vi "SimulationEngine-Media.vi"(0 "Use Slab Geometry (F: Sphere)":bool, 1 "File Prefix":string, 4 "Simulation Grain (mm)":dbl=0.0001, 5 "Radius (mm)":dbl=5.0, 6 "N Photons":i32=1, 7 "Starting Depth (mm)":dbl=2.0, 8 "G":dbl=nan, 9 "Absorption Coefficient":dbl=0.00645, 10 "Scattering Coefficient":dbl=1.688, 11 "folder path":path) -> (2 "Diagram":cluster{dbl[], dbl[]}[](graph), 3 "new file path (Not A Path if cancelled)":path)   [LabVIEW 2019]
uses:
  <vilib>/Utility/file.llb/Write Delimited Spreadsheet (string).vi
panel:
  out "Numeric":i32
  out "dT":dbl
  out "Current Index":i32
  # "18.638"
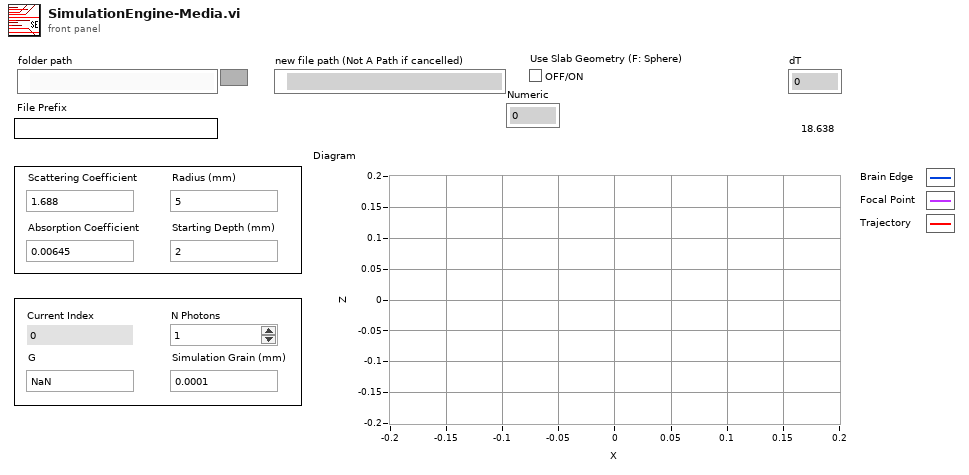
[diagram p1: front panel]
types:
  T1 = cluster{"Starting Depth":dbl, "Starting Depth":dbl, dbl}
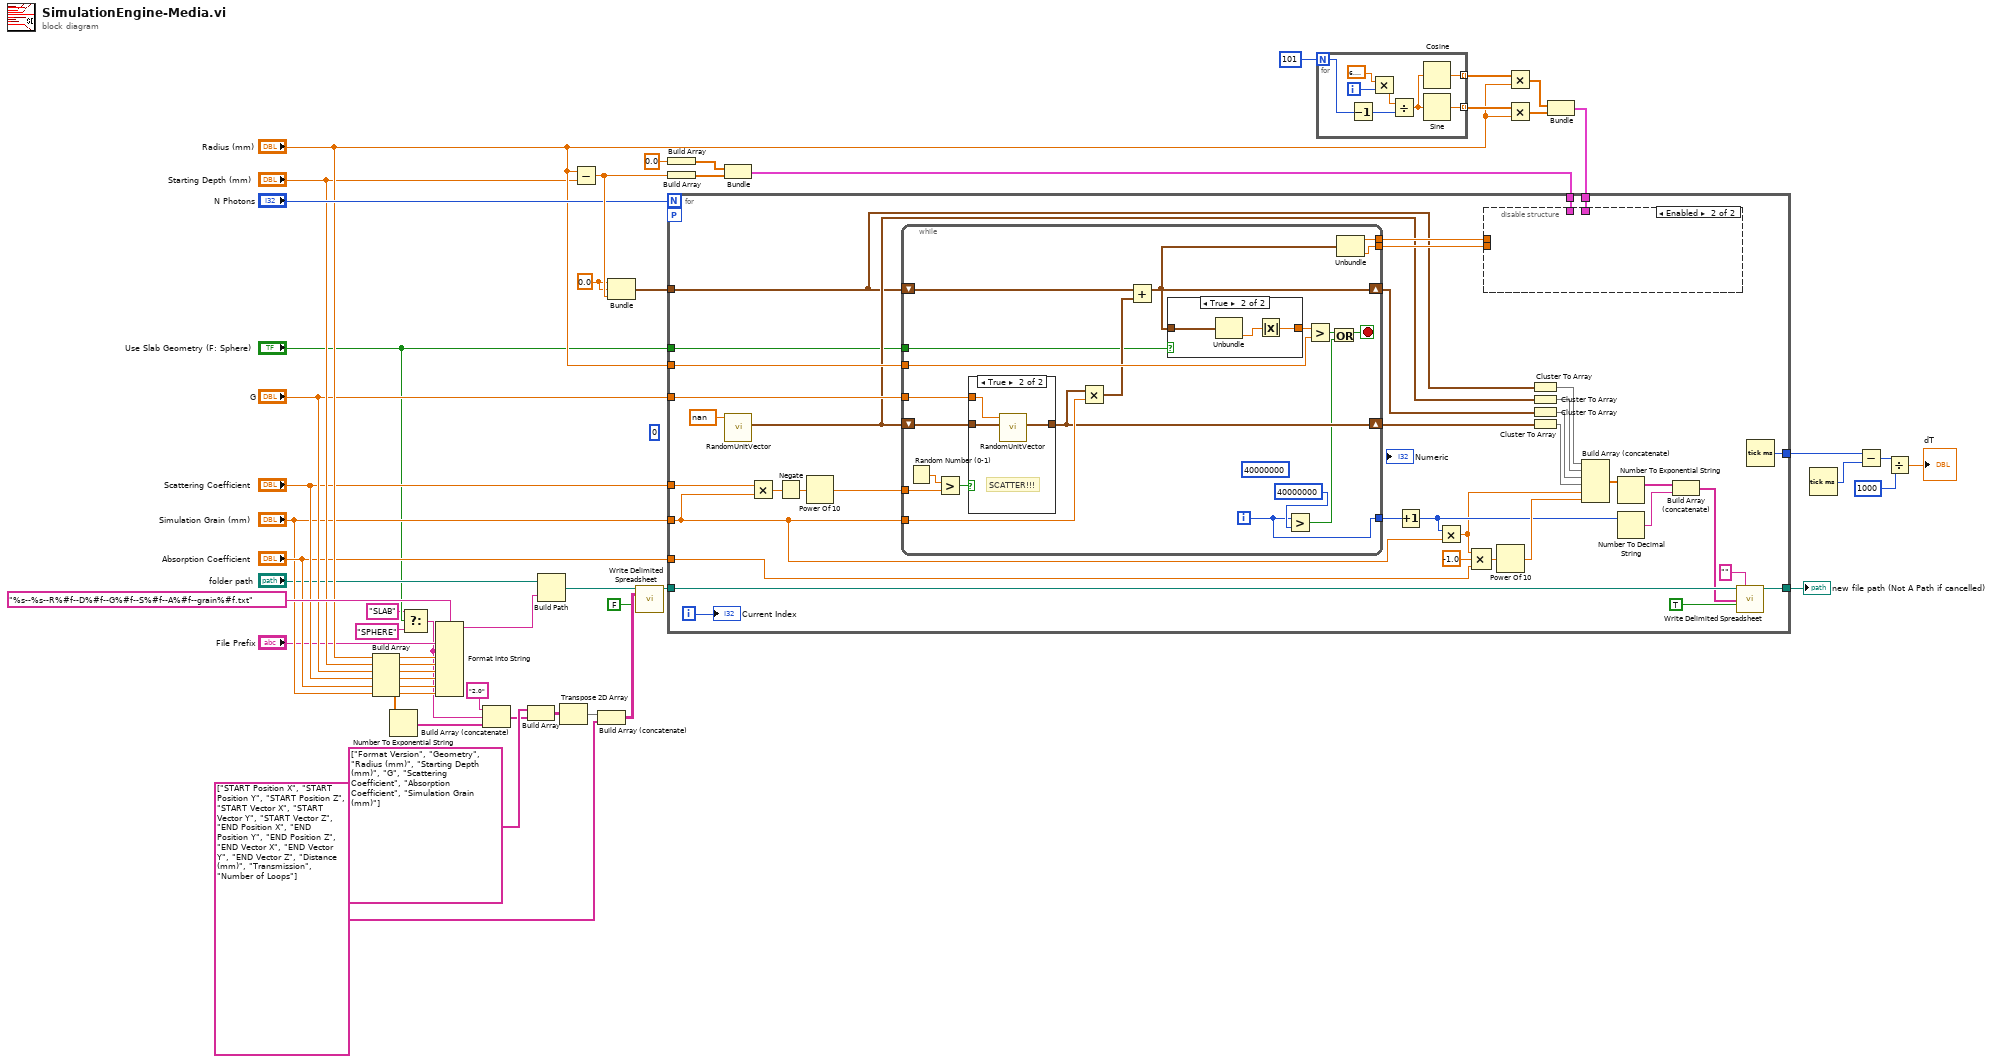
[diagram p0: block diagram]
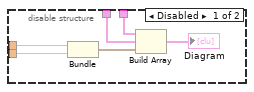
[diagram p2: hidden frame]
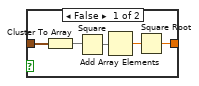
[diagram p3: hidden frame]
diagram:
  (unwired) 0
  w42 = 0.0 ("Starting Depth")
  n1 = Build Array("Radius (mm)", "Starting Depth (mm)", "G", "Scattering Coefficient", "Absorption Coefficient", "Simulation Grain (mm)") -> (w30:dbl[])
  n2 = Number To Exponential String(number=w30) -> (E-format string=w28:string[])  [unwired: 3 in]
  n3 = Select(t="SLAB" ("format string"), s="Use Slab Geometry (F: Sphere)", f="SPHERE" ("format string")) -> (s? t:f=w6:string)
  n4 = Format Into String(format string="%s--%s--R%#f--D%#f--G%#f--S%#f--A%#f--grain%#f.txt", "File Prefix", w6, "Radius (mm)", "Starting Depth (mm)", "G", "Scattering Coefficient", "Absorption Coefficient", "Simulation Grain (mm)") -> (resulting string=w13:string)  [unwired: 2 in, 1 out]
  n5 = Build Array (concatenate)("2.0" ("Simulation Grain (mm)"), w6, w28) -> (w8:string[])
  n6 = Build Array(string[] ["Format Version", "Geometry", "Radius (mm)", "Starting Depth (mm)", "G", "Scattering Coefficient", "Absorption Coefficient", "Simulation Grain (mm)"] ("E-format string"), w8) -> (w27:string[][])
  n7 = Build Path(base path="folder path", name or relative path=w13) -> (appended path=w14:path)
  n8 = Transpose 2D Array(2D array=w27) -> (transposed array=w26:string[][])
  n9 = Subtract(x="Radius (mm)", y="Starting Depth (mm)") -> (x-y=w43:dbl)
  n10 = Build Array (concatenate)(w26, string[] ["START Position X", "START Position Y", "START Position Z", "START Vector X", "START Vector Y", "START Vector Z", "END Position X", "END Position Y", "END Position Z", "END Vector X", "END Vector Y", "END Vector Z", "Distance (mm)", "Transmission", "Number of Loops"] ("E-format string")) -> (w24:string[][])
  n11 = Bundle("Starting Depth"=w42, "Starting Depth"=w42, w43) -> (w44:T1)  [unwired: 1 in]
  n12 = call-poly <vilib>:"Write Delimited Spreadsheet.vi"("file path (dialog if empty)"=w14, "2D data"=w24, "append to file? (new file:F)"=FALSE) -> ("new file path (Not A Path if cancelled)"=w31:path)  [unwired: 11 in, 1 out]
  n13 = Build Array(0.0 ("Starting Depth")) -> (w40:dbl[])
  n14 = Build Array(w43) -> (w39:dbl[])
  n15 = Bundle(w40, w39) -> (w45:cluster{dbl[], dbl[]})  [unwired: 1 in]
  n16 = for {
    N: 101 -> [w51]
    tunnel: [w49] -> w36 mode=indexing
    tunnel: [w47] -> w35 mode=indexing
    i -> [w54]
    n17 = Decrement(x=w51) -> (x-1=w50:i32)
    n18 = Multiply(x=6.283185307179586, y=w54) -> (x*y=w52:dbl)
    n19 = Divide(x=w52, y=w50) -> (x/y=w48:dbl)
    n20 = Cosine(x=w48) -> (cos(x)=w47:dbl)
    n21 = Sine(x=w48) -> (sin(x)=w49:dbl)
  }
  n22 = Multiply(x=w35, y="Radius (mm)") -> (x*y=w37:dbl[])
  n23 = Multiply(x=w36, y="Radius (mm)") -> (x*y=w38:dbl[])
  n24 = Bundle(w37, w38) -> (w46:cluster{dbl[], dbl[]})  [unwired: 1 in]
  n25 = for {
    N: "N Photons" -> [_]
    tunnel: "Radius (mm)" -> [w90]
    tunnel: "Scattering Coefficient" -> [w87]
    tunnel: "Absorption Coefficient" -> [w58]
    tunnel: "Simulation Grain (mm)" -> [w61]
    tunnel: w44 -> [w70]
    tunnel: w45 -> [w85]
    tunnel: w46 -> [w84]
    tunnel: "G" -> [w72]
    tunnel: "Use Slab Geometry (F: Sphere)" -> [w69]
    tunnel: w31 -> [w83]
    tunnel: [w82] -> w33
    tunnel: [w56] -> w5
    workers-P: _ -> [_]
    i -> [w81]
    n26 = call "RandomUnitVector.vi"("G"=nan) -> ("Random 3D Unit Vector"=w71:cluster{"X":dbl, "Y":dbl, "Z":dbl})  [unwired: 9 in, 1 out]
    n27 = Multiply(x=w87, y=w61) -> (x*y=w88:dbl)
    n28 = Negate(x=w88) -> (-x=w89:dbl)
    n29 = Power Of 10(x=w89) -> (10^x=w86:dbl)
    n30 = while {
      shift-right: [w103] -> w74
      shift-left: w70 -> [w115]
      tunnel: [w107] -> w92
      tunnel: [w106] -> w91
      tunnel: w90 -> [w117]
      shift-right: [w109] -> w78
      shift-left: w71 -> [w110]
      tunnel: w61 -> [w114]
      tunnel: w86 -> [w113]
      tunnel: w72 -> [w105]
      tunnel: w69 -> [w104]
      tunnel: [w99] -> w55
      i -> [w99]
      stop <- w101 stop-if-true
      (unwired) 40000000
      n31 = Random Number (0-1)() -> (number: 0 to 1=w112:dbl)
      n32 = Greater?(x=w112, y=w113) -> (0:w111:bool)
      n33 = case shown="True" w111 {
        tunnel: w110 -> [w127 w128]
        tunnel: [w127 w130] -> w109
        tunnel: w105 -> [_ w129]
        frame False {
        }
        frame True {
          # "SCATTER!!!"
          n34 = call "RandomUnitVector.vi"("Old 3D Unit Vector"=w128, "G"=w129) -> ("Random 3D Unit Vector"=w130:cluster{"X":dbl, "Y":dbl, "Z":dbl})  [unwired: 8 in, 1 out]
        }
      }
      n35 = Multiply(x=w109, y=w114) -> (x*y=w108:cluster{"X":dbl, "Y":dbl, "Z":dbl})
      n36 = Add(x=w115, y=w108) -> (x+y=w103:cluster{dbl, dbl, dbl})
      n37 = case shown="True" w104 {
        tunnel: [w121 w124] -> w118
        tunnel: w103 -> [w120 w126]
        frame False {
          n38 = Cluster To Array(cluster=w120) -> (array=w119:dbl[])
          n39 = Square(x=w119) -> (x^2=w123:dbl[])
          n40 = Add Array Elements(numeric array=w123) -> (sum=w122:dbl)
          n41 = Square Root(x=w122) -> (sqrt(x)=w121:dbl)
        }
        frame True {
          n42 = Unbundle(w126) -> (w125:dbl)  [unwired: 2 out]
          n43 = Absolute Value(x=w125) -> (abs(x)=w124:dbl)
        }
      }
      n44 = Greater?(x=w99, y=40000000) -> (0:w100:bool)
      n45 = Greater?(x=w118, y=w117) -> (0:w116:bool)
      n46 = Or(x=w116, y=w100) -> (x .or. y?=w101:bool)
      n47 = Unbundle(w103) -> (w107:dbl, w106:dbl)  [unwired: 1 out]
    }
    n48 = Increment(x=w55) -> (x+1=w60:i32)
    n49 = Multiply(x=w60, y=w61) -> (x*y=w59:dbl)
    n50 = Compound Arithmetic op=MULTIPLY(w59, -1.0 ("value"), w58) -> (w65:dbl)
    n51 = disable-structure shown="Enabled" {
      disable-tunnel: w92 -> [w98 _]
      disable-tunnel: w91 -> [w97 _]
      disable-tunnel: w85 -> [w94 _]
      disable-tunnel: w84 -> [w93 _]
      frame Disabled {
        n52 = Bundle(w98, w97) -> (w95:cluster{dbl, dbl})  [unwired: 1 in]
        n53 = Build Array(w93, w94, w95) -> (→"Diagram":cluster{dbl[], dbl[]}[])
      }
      frame Enabled {
      }
    }
    n54 = Power Of 10(x=w65) -> (10^x=w62:dbl)
    n55 = Cluster To Array(cluster=w70) -> (array=w64:dbl[])
    n56 = Cluster To Array(cluster=w71) -> (array=w63:dbl[])
    n57 = Cluster To Array(cluster=w74) -> (array=w77:dbl[])
    n58 = Cluster To Array(cluster=w78) -> (array=w76:dbl[])
    n59 = Build Array (concatenate)(w64, w63, w77, w76, w59, w62) -> (w75:dbl[])
    n60 = Number To Exponential String(number=w75) -> (E-format string=w67:string[])  [unwired: 3 in]
    n61 = Number To Decimal String(number=w60) -> (decimal integer string=w68:string)  [unwired: 1 in]
    n62 = Build Array (concatenate)(w67, w68) -> (w66:string[])
    n63 = call-poly <vilib>:"Write Delimited Spreadsheet.vi"("file path (dialog if empty)"=w83, "format (%s)"="" ("format (%.3f)"), "1D data"=w66, "append to file? (new file:F)"=TRUE) -> ("new file path (Not A Path if cancelled)"=w82:path)  [unwired: 10 in, 1 out]
    n64 = Tick Count (ms)() -> (millisecond timer value=w56:u32)
    "Current Index" <- w81
  }
  "new file path (Not A Path if cancelled)" <- w33
  n65 = Tick Count (ms)() -> (millisecond timer value=w4:u32)
  n66 = Subtract(x=w5, y=w4) -> (x-y=w3:u32)
  n67 = Divide(x=w3, y=u32 1000) -> (x/y=→"dT":dbl)
